vi "Configure Output.vi"(6 "Frequency (50 Hz)":dbl=50.0 min=43.0 max=1200.0 format="%.3g", 8 "error in (no error)":errorcluster, 9 "DC Voltage Level (0.0 V)":dbl format="%.3g", 10 "AC Voltage Level (0.0 V)":dbl format="%.3g", 11 "VISA resource name":refnum<visa-resource-name>) -> (0 "error out":errorcluster, 3 "VISA resource name out":refnum<visa-resource-name>)   [LabVIEW 2015, in "BK Precision 983X Series.lvlib"]
doc: "Configures output AC and DC voltage levels and frequency."
uses:
  <instrlib>/BK Precision 983X Series/BK Precision 983X Series.lvlib
panel:
  # "Hz"
  # "V"
  # "V"
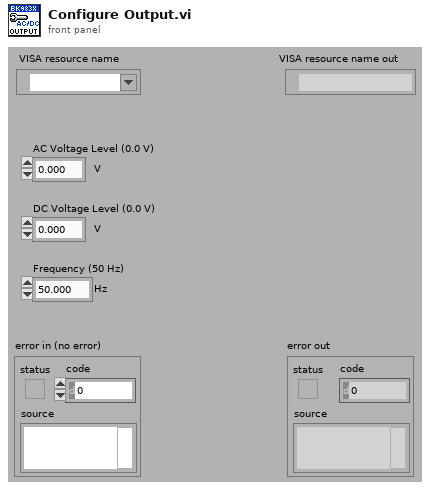
[diagram p1: front panel]
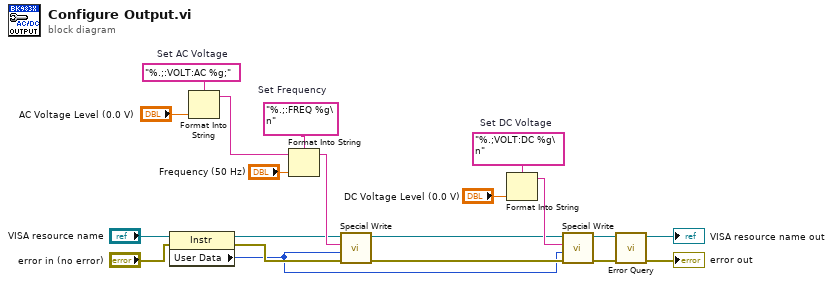
[diagram p0: block diagram]
diagram:
  w13 = "%.;:FREQ %g\n"  # Set Frequency
  w14 = "%.;VOLT:DC %g\n"  # Set DC Voltage
  w18 = "%.;:VOLT:AC %g;"  # Set AC Voltage
  n1 = property class="Instr"(reference="VISA resource name", error in="error in (no error)") -> (reference out=w9:refnum<visa-resource-name>, error out=w8:errorcluster, "User Data"=w3:u32)
  n2 = Format Into String(format string=w18, "AC Voltage Level (0.0 V)") -> (resulting string=w7:string)  [unwired: 2 in, 1 out]
  n3 = Format Into String(format string=w13, initial string=w7, "Frequency (50 Hz)") -> (resulting string=w10:string)  [unwired: 1 in, 1 out]
  n4 = call <instrlib>:"Special Write.vi"("error in (no error)"=w8, "Delay (0 ms)"=w3, "Input String"=w10, "VISA resource name"=w9) -> ("error out"=w4:errorcluster, "VISA resource name out"=w1:refnum<visa-resource-name>)  [unwired: 6 in]
  n5 = Format Into String(format string=w14, "DC Voltage Level (0.0 V)") -> (resulting string=w2:string)  [unwired: 2 in, 1 out]
  n6 = call <instrlib>:"Special Write.vi"("error in (no error)"=w4, "Delay (0 ms)"=w3, "Input String"=w2, "VISA resource name"=w1) -> ("error out"=w5:errorcluster, "VISA resource name out"=w6:refnum<visa-resource-name>)  [unwired: 6 in]
  n7 = call <instrlib>:"Error Query.vi"("error in (no error)"=w5, "VISA resource name"=w6) -> ("error out"=→"error out":errorcluster, "VISA resource name out"=→"VISA resource name out":refnum<visa-resource-name>)  [unwired: 6 in, 2 out]
